vi "UHR-Fleezers Control (host) - 12.0.vi"() -> ()   [LabVIEW 2012] (continued)
        n1597 = case shown="True" w2753 {
          tunnel: [w2765 1] -> w2754
          tunnel: w2758 -> [w2767 _]
          tunnel: [w2766 w2785] -> w2755
          tunnel: w2756 -> [w2766 _]
          tunnel: w2752 -> [_ w2805]
          tunnel: w2745 -> [_ w2803]
          tunnel: w2747 -> [_ w2806]
          tunnel: [w2764 w2784] -> w2744
          tunnel: w2746 -> [w2764 _]
          tunnel: [w2763 w2782] -> w2741
          tunnel: w2742 -> [w2763 _]
          tunnel: [w2762 w2781] -> w2738
          tunnel: w2739 -> [w2762 _]
          tunnel: "Start Saving" -> [_ w2779]
          tunnel: w2734 -> [_ w2778]
          tunnel: [w2761 w2769] -> w2727
          tunnel: w2731 -> [w2761 _]
          tunnel: [w2760 w2768] -> w2728
          tunnel: w2729 -> [w2760 _]
          frame False {
            n1598 = Increment(x=w2767) -> (x+1=w2765:i32)
          }
          frame True {
            w2775 = FALSE ("Start Saving")
            w2780 = 9.0  # File Version
            w2788 = FALSE ("prepend array or string size? (T)")
            w2786 = T36."big-endian, network order" ("byte order (0:big-endian, network order)")
            n1599 = local read "BD 1 Frequency 1 (MHz)"() -> (w2802:dbl)
            n1600 = local read "BD 2 Frequency 1 (MHz)"() -> (w2801:dbl)
            n1601 = local read "BD 1 Frequency 2 (MHz)"() -> (w2800:dbl)
            n1602 = local read "BD 2 Frequency 2 (MHz)"() -> (w2799:dbl)
            n1603 = local read "BD 1 Frequency 3 (MHz)"() -> (w2798:dbl)
            n1604 = local read "BD 2 Frequency 3 (MHz)"() -> (w2797:dbl)
            n1605 = Array Size(array=w2778) -> (size(s)=w2777:i32)
            n1606 = To Double Precision Float(number=w2777) -> (double precision float=w2776:dbl)
            n1607 = local write "Save Calibration"(w2775) -> ()
            n1608 = local write "Start Saving"(w2775) -> ()
            n1609 = Build Array("Save APD Data\nwith Trap Data", "Save Trap Pos. Data") -> (w2772:bool[])
            n1610 = Boolean Array To Number(Boolean array=w2772) -> (number=w2771:u32)
            n1611 = Build Array(w2802, w2801, w2800, w2799, w2798, w2797) -> (w2796:dbl[])
            n1612 = case shown="1, Default" w2806 {
              tunnel: w2805 -> [w2877 w2897 w2913 w2951]
              tunnel: w2776 -> [w2882 w2904 w2933 w2970]
              tunnel: w2803 -> [w2881 w2903 w2932 w2969]
              tunnel: [w2878 w2899 w2924 w2961] -> w2794
              tunnel: [w2869 "Cal sets to save" w2914 w2952] -> w2784
              tunnel: w2796 -> [w2879 w2900 w2926 w2963]
              tunnel: "Save APD Data\nwith Trap Data" -> [w2876 _ w2910 w2949]
              tunnel: [w2876 w2891 w2910 w2949] -> w2781
              tunnel: w2780 -> [w2872 w2892 w2908 w2947]
              tunnel: w2779 -> [w2871 _ _ _]
              tunnel: [w2862 w2891 w2907 w2937] -> w2768
              tunnel: "Save Trap Pos. Data" -> [w2862 _ w2907 w2937]
              tunnel: w2771 -> [w2861 _ w2906 w2936]
              frame 1, Default {
                # "timeseries"
                n1613 = case shown="True" "Profile" {
                  tunnel: [w2885 w2889] -> w2866
                  tunnel: [w2885 w2888] -> w2865
                  tunnel: [w2885 w2887] -> w2864
                  tunnel: [w2885 w2886] -> w2863
                  frame False {
                    w2885 = 0.0 ("f")
                  }
                  frame True {
                    n1614 = local read "Current Position"() -> (w2890:cluster{dbl, dbl, dbl})
                    n1615 = local read "Y change (mm)"() -> (w2886:dbl)
                    n1616 = Unbundle(w2890) -> (w2889:dbl, w2888:dbl, w2887:dbl)
                  }
                }
                n1617 = local read "Save ave N"() -> (w2884:dbl)
                n1618 = Multiply(x=w2884, y=w2877) -> (x*y=w2883:dbl)
                n1619 = To Double Precision Float(number=w2861) -> (double precision float=w2875:dbl)
                n1620 = Build Array(w2872, w2877, w2883, w2882, w2881, 0.0 ("f")) -> (w2880:dbl[])
                n1621 = Build Array(w2875, w2866, w2865, w2864, w2863) -> (w2873:dbl[])
                n1622 = Select(t=u32 4000000000, s=w2871, f="N sets to save") -> (s? t:f=w2869:u32)
                n1623 = Build Array (concatenate)(w2880, w2879, w2873) -> (w2878:dbl[])
              }
              frame 2 {
                w2894 = 0.0 ("f")
                w2891 = FALSE ("Save APD Data\nwith Trap Data")
                # "calibration"
                n1624 = Boolean To (0,1)(Boolean=w2891) -> (0, 1=w2896:i16)
                n1625 = To Double Precision Float(number=w2896) -> (double precision float=w2895:dbl)
                n1626 = Build Array(w2895, w2894, w2894, w2894, w2894) -> (w2893:dbl[])
                n1627 = Build Array(w2892, w2897, w2897, w2904, w2903, 1.0 ("t")) -> (w2901:dbl[])
                n1628 = Build Array (concatenate)(w2901, w2900, w2893) -> (w2899:dbl[])
                "Calibrating Trap..." <- TRUE ("Calibrating...")
              }
              frame 4 {
                w2911 = 0.0 ("f")
                # "scan dir (x/y = 0/1)"
                # "cycles/step"
                # "n scans (f/b)"
                # "steps"
                # "freq. range"
                # "AOD raster scan"
                n1629 = local read "Number of F/B Scans (AOD)"() -> (w2918:u16)
                n1630 = local read "Cycles/step (AOD)"() -> (w2920:u64)
                n1631 = local read "Scan Range (MHz)"() -> (w2923:dbl)
                n1632 = local read "Scan steps (AOD)"() -> (w2922:u64)
                n1633 = local read "Scan BD"() -> (w2930:bool)
                n1634 = local read "Save ave N"() -> (w2935:dbl)
                n1635 = Boolean To (0,1)(Boolean=w2930) -> (0, 1=w2929:i16)
                n1636 = To Double Precision Float(number=w2918) -> (double precision float=w2917:dbl)
                n1637 = To Double Precision Float(number=w2922) -> (double precision float=w2921:dbl)
                n1638 = To Double Precision Float(number=w2920) -> (double precision float=w2919:dbl)
                n1639 = To Double Precision Float(number=w2929) -> (double precision float=w2928:dbl)
                n1640 = Multiply(x=w2935, y=w2913) -> (x*y=w2934:dbl)
                n1641 = To Double Precision Float(number=w2906) -> (double precision float=w2912:dbl)
                n1642 = Build Array(w2912, w2911, w2911, w2911, w2911) -> (w2909:dbl[])
                n1643 = local read "N sets should be saved"() -> (w2915:dbl)
                n1644 = Build Array(w2928, w2923, w2921, w2919, w2917) -> (w2925:dbl[])
                n1645 = Build Array(w2908, w2913, w2934, w2933, w2932, 2.0 ("t")) -> (w2927:dbl[])
                n1646 = Round Toward +Infinity(x=w2915) -> (ceil(x): smallest int >= x=w2916:dbl)
                n1647 = Build Array (concatenate)(w2927, w2926, w2909, w2925) -> (w2924:dbl[])
                n1648 = To Unsigned Long Integer(number=w2916) -> (unsigned 32bit integer=w2914:u32)
              }
              frame 8 {
                w2944 = 0.0 ("f")
                # "MCL raster scan"
                n1649 = local read "Number of scans (MCL)"() -> (w2939:u64)
                n1650 = local read "Scan lines (y)"() -> (w2938:u64)
                n1651 = local read "2D or 1D Scan"() -> (w2941:bool)
                n1652 = local read "Scan Range (V)\n(of steps)"() -> (w2960:dbl)
                n1653 = local read "Fast Scan Dir"() -> (w2967:bool)
                n1654 = local read "Cycles/step (MCL)"() -> (w2957:u64)
                n1655 = local read "Scan steps (MCL)"() -> (w2959:u64)
                n1656 = Select(t=w2938, s=w2941, f=w2939) -> (s? t:f=w2940:u64)
                n1657 = Boolean To (0,1)(Boolean=w2941) -> (0, 1=w2943:i16)
                n1658 = local read "Save ave N"() -> (w2972:dbl)
                n1659 = local read "Initial X"() -> (w2946:dbl)
                n1660 = local read "Initial Y"() -> (w2945:dbl)
                n1661 = To Double Precision Float(number=w2943) -> (double precision float=w2942:dbl)
                n1662 = Boolean To (0,1)(Boolean=w2967) -> (0, 1=w2966:i16)
                n1663 = To Double Precision Float(number=w2940) -> (double precision float=w2955:dbl)
                n1664 = To Double Precision Float(number=w2959) -> (double precision float=w2958:dbl)
                n1665 = To Double Precision Float(number=w2957) -> (double precision float=w2956:dbl)
                n1666 = To Double Precision Float(number=w2966) -> (double precision float=w2965:dbl)
                n1667 = Multiply(x=w2972, y=w2951) -> (x*y=w2971:dbl)
                n1668 = To Double Precision Float(number=w2936) -> (double precision float=w2950:dbl)
                n1669 = local read "N sets should be saved (MCL)"() -> (w2953:dbl)
                n1670 = Build Array(w2950, w2942, w2944, w2944, w2944) -> (w2948:dbl[])
                n1671 = Build Array(w2965, w2960, w2958, w2956, w2955, w2946, w2945) -> (w2962:dbl[])
                n1672 = Build Array(w2947, w2951, w2971, w2970, w2969, 3.0 ("t")) -> (w2964:dbl[])
                n1673 = Round Toward +Infinity(x=w2953) -> (ceil(x): smallest int >= x=w2954:dbl)
                n1674 = Build Array (concatenate)(w2964, w2963, w2948, w2962) -> (w2961:dbl[])
                n1675 = To Unsigned Long Integer(number=w2954) -> (unsigned 32bit integer=w2952:u32)
              }
            }
            n1676 = local read "Index"() -> (w2811:dbl)
            n1677 = call "Create new save file.vi"("Insert"="", "Ext"=".dat", "Index In"=w2811) -> ("Path Out"=w2770:path, "Index Out"=w2783:dbl)
            n1678 = local write "Save file name"(w2770) -> ()
            n1679 = local write "Index"(w2783) -> ()
            n1680 = local write "Save index"(w2783) -> ()
            n1681 = Array Size(array=w2794) -> (size(s)=w2795:i32)
            n1682 = Open/Create/Replace File(file path (use dialog)=w2770, operation (0:open)=T35."create", access (0:read/write)=enum16{"read/write", "read-only", "write-only"}."write-only") -> (refnum out=w2808:refnum<file>)  [unwired: 1 in, 4 out]
            n1683 = local write "Saving..."(TRUE ("Saving...")) -> ()
            n1684 = To Double Precision Float(number=w2795) -> (double precision float=w2793:dbl)
            n1685 = String Length(string="Comment (data description)") -> (length=w2791:i32)
            n1686 = To Double Precision Float(number=w2791) -> (double precision float=w2790:dbl)
            n1687 = Deny Access(7:w2808) -> (3:w2807:refnum<file>)  [unwired: 1 in, 2 out]
            n1688 = Build Array (concatenate)(w2793, w2794, w2790) -> (w2792:dbl[])
            n1689 = case "If fluorescence data to be saved" shown="True" w2781 {
              tunnel: w2770 -> [_ w2860]
              tunnel: [refnum<k0> refnum w2840] -> w2782
              frame False {
              }
              frame True {
                w2839 = 0.0
                n1690 = local read "APD Integration Time (s)"() -> (w2845:dbl)
                n1691 = local read "N APD Samp/step"() -> (w2838:dbl)
                n1692 = Path To String(path=w2860) -> (string=w2859:string)
                n1693 = String Length(string=w2859) -> (length=w2858:i32)
                n1694 = Subtract(x=w2858, y=4) -> (x-y=w2856:i32)
                n1695 = String Subset(string=w2859, length (rest)=w2856) -> (substring=w2855:string)  [unwired: 1 out]
                n1696 = Build Array(w2845, w2838, w2839, w2839, w2839, w2839, w2839, w2839) -> (w2842:dbl[])
                n1697 = Concatenate Strings(w2855, "_fl.dat" ("string")) -> (w2853:string)
                n1698 = Array Size(array=w2842) -> (size(s)=w2844:i32)
                n1699 = String To Path(string=w2853) -> (path=w2849:path)
                n1700 = Open/Create/Replace File(file path (use dialog)=w2849, operation (0:open)=T35."create", access (0:read/write)=enum16{"read/write", "read-only", "write-only"}."write-only") -> (refnum out=w2850:refnum<file>)  [unwired: 1 in, 4 out]
                n1701 = Deny Access(7:w2850) -> (3:w2846:refnum<file>)  [unwired: 1 in, 2 out]
                n1702 = To Double Precision Float(number=w2844) -> (double precision float=w2843:dbl)
                n1703 = Build Array (concatenate)(w2843, w2842) -> (w2841:dbl[])
                n1704 = Write to Binary File(file (use dialog)=w2846, data=w2841, 5:FALSE ("prepend array or string size? (T)"), 9:T36."big-endian, network order" ("byte order (0:big-endian, network order)")) -> (refnum out=w2840:refnum<file>)  [unwired: 1 in, 3 out]
              }
            }
            n1705 = case shown="True" w2768 {
              tunnel: w2770 -> [_ w2822]
              tunnel: [refnum<k0> refnum w2821] -> w2769
              frame False {
              }
              frame True {
                w2817 = 0.0 ("element")
                n1706 = Path To String(path=w2822) -> (string=w2836:string)
                n1707 = Build Array(w2817, w2817, w2817, w2817, w2817, w2817, w2817, w2817) -> (w2818:dbl[])
                n1708 = String Length(string=w2836) -> (length=w2835:i32)
                n1709 = Subtract(x=w2835, y=4) -> (x-y=w2833:i32)
                n1710 = Array Size(array=w2818) -> (size(s)=w2820:i32)
                n1711 = String Subset(string=w2836, length (rest)=w2833) -> (substring=w2832:string)  [unwired: 1 out]
                n1712 = To Double Precision Float(number=w2820) -> (double precision float=w2819:dbl)
                n1713 = Concatenate Strings(w2832, "_pos.dat" ("string")) -> (w2830:string)
                n1714 = Build Array (concatenate)(w2819, w2818) -> (w2816:dbl[])
                n1715 = String To Path(string=w2830) -> (path=w2826:path)
                n1716 = Open/Create/Replace File(file path (use dialog)=w2826, operation (0:open)=T35."create", access (0:read/write)=enum16{"read/write", "read-only", "write-only"}."write-only") -> (refnum out=w2827:refnum<file>)  [unwired: 1 in, 4 out]
                n1717 = Deny Access(7:w2827) -> (3:w2823:refnum<file>)  [unwired: 1 in, 2 out]
                n1718 = Write to Binary File(file (use dialog)=w2823, data=w2816, 5:FALSE ("prepend array or string size? (T)"), 9:T36."big-endian, network order" ("byte order (0:big-endian, network order)")) -> (refnum out=w2821:refnum<file>)  [unwired: 1 in, 3 out]
              }
            }
            n1719 = Write to Binary File(file (use dialog)=w2807, data=w2792, 5:w2788, 9:w2786) -> (refnum out=w2789:refnum<file>)  [unwired: 1 in, 3 out]
            n1720 = Write to Binary File(file (use dialog)=w2789, data="Comment (data description)", 5:w2788, 9:w2786) -> (refnum out=w2785:refnum<file>)  [unwired: 1 in, 3 out]
          }
        }
        n1721 = feedback-in #28(w2728) -> ()
        n1722 = feedback-in #29(w2755) -> ()
        n1723 = feedback-in #30(w2727) -> ()
        n1724 = feedback-in #31(w2738) -> ()
        n1725 = feedback-in #32(w2741) -> ()
        n1726 = feedback-in #33(w2754) -> ()
        n1727 = feedback-in #34(w2744) -> ()
      }
      frame #1 {
        n1728 = local read "Saving..."() -> (w2986:bool)
        n1729 = case shown="True" w2986 {
          tunnel: w2990 -> [_ w3001]
          tunnel: w2989 -> [_ w3015]
          tunnel: w2988 -> [_ w3011]
          tunnel: w2987 -> [_ w3010]
          tunnel: w2985 -> [_ w3009]
          tunnel: w2984 -> [_ w3004]
          tunnel: w2983 -> [_ w3003]
          tunnel: w2982 -> [_ w3002]
          tunnel: w2981 -> [_ w3000]
          tunnel: w2980 -> [_ w2998]
          tunnel: w2979 -> [_ w2997]
          tunnel: w2978 -> [_ w2996]
          tunnel: w2977 -> [_ w2995]
          tunnel: w2976 -> [_ w2994]
          tunnel: w2975 -> [_ w2993]
          tunnel: w2974 -> [_ w2992]
          tunnel: w2973 -> [_ w2991]
          frame False {
          }
          frame True {
            n1730 = Multiply(x=w3001, y=w3000) -> (x*y=→"Time (s)":dbl)
            n1731 = Less Or Equal?(x=w3001, y=w3009) -> (x <= y?=w3013:bool)
            n1732 = Or(x="Stop Saving", y="Abort save 2") -> (x .or. y?=w3005:bool)
            n1733 = Not(x=w3005) -> (.not. x?=w3014:bool)
            n1734 = And(x=w3013, y=w3014) -> (x .and. y?=w3012:bool)
            n1735 = case shown="True" w3012 {
              tunnel: w3015 -> [w3022 w3097]
              tunnel: [0.0 w3100] -> w3008
              tunnel: w3001 -> [_ w3098]
              tunnel: w3009 -> [_ w3099]
              tunnel: w3011 -> [_ w3094]
              tunnel: w3010 -> [_ _]
              tunnel: w3004 -> [w3020 w3087]
              tunnel: w3003 -> [w3019 w3088]
              tunnel: w3002 -> [_ w3086]
              tunnel: w2998 -> [_ w3085]
              tunnel: w2997 -> [_ w3029]
              tunnel: w2996 -> [_ w3078]
              tunnel: w2995 -> [_ w3056]
              tunnel: w2994 -> [w3016 w3038]
              tunnel: w2993 -> [w3017 w3037]
              tunnel: w2992 -> [_ w3034]
              tunnel: w2991 -> [_ w3032]
              frame False {
                w3018 = FALSE
                n1736 = Close File(refnum=w3022) -> ()  [unwired: 1 in, 2 out]
                n1737 = case shown="True" w3019 {
                  tunnel: w3020 -> [_ w3024]
                  frame False {
                  }
                  frame True {
                    n1738 = Close File(refnum=w3024) -> ()  [unwired: 1 in, 2 out]
                  }
                }
                n1739 = case shown="True" w3016 {
                  tunnel: w3017 -> [_ w3023]
                  frame False {
                  }
                  frame True {
                    n1740 = Close File(refnum=w3023) -> ()  [unwired: 1 in, 2 out]
                  }
                }
                n1741 = local write "Raster Scanning..."(w3018) -> ()
                n1742 = local write "Calibrating Trap..."(w3018) -> ()
                n1743 = call <vilib>:"Beep.vi"() -> ()  [unwired: 3 in, 9 out]
                n1744 = local write "Stop Saving"(w3018) -> ()
                "Saving..." <- w3018
              }
              frame True {
                n1745 = local read "Calibrating Trap..."() -> (w3089:bool)
                n1746 = case "Write fl. data" shown="True" w3088 {
                  tunnel: w3087 -> [_ w3123]
                  tunnel: w3086 -> [_ w3122]
                  frame False {
                  }
                  frame True {
                    n1747 = Write to Binary File(file (use dialog)=w3123, data=w3122, 5:FALSE ("prepend array or string size? (T)"), 9:T36."big-endian, network order" ("byte order (0:big-endian, network order)")) -> ()  [unwired: 1 in, 4 out]
                  }
                }
                n1748 = Greater?(x="Save ave N", y=1.0) -> (0:w3092:bool)
                n1749 = Not(x=w3089) -> (.not. x?=w3091:bool)
                n1750 = And(x=w3091, y=w3092) -> (x .and. y?=w3035:bool)
                n1751 = case shown="True" w3035 {
                  tunnel: w3034 -> [w3103 w3114]
                  tunnel: [w3103 w3106] -> w3033
                  tunnel: "Save ave N" -> [_ w3107]
                  frame False {
                  }
                  frame True {
                    w3104 = 2 ("dimension size")
                    n1752 = Array Size(array=w3114) -> (size(s)=w3108:i32)
                    n1753 = Divide(x=w3108, y=w3104) -> (x/y=w3112:dbl)
                    n1754 = Reshape Array(w3114, w3112, w3104) -> (w3113:u64[][])
                    n1755 = Transpose 2D Array(2D array=w3113) -> (transposed array=w3111:u64[][])
                    n1756 = for {
                      tunnel: w3111 -> [w3116] mode=indexing
                      tunnel: [w3115] -> w3105 mode=indexing
                      tunnel: w3107 -> [w3117]
                      workers-P: _ -> [_]
                      n1757 = call "downsample 1D array - U64.vi"("Ave N"=w3117, "Array In"=w3116) -> ("Array Out"=w3115:u64[])  [unwired: 1 in]
                    }
                    n1758 = Transpose 2D Array(2D array=w3105) -> (transposed array=w3110:u64[][])
                    n1759 = Divide(x=w3108, y=w3107) -> (x/y=w3109:dbl)
                    n1760 = Reshape Array(w3110, w3109) -> (w3106:u64[])
                  }
                }
                n1761 = case shown="True" w3035 {
                  tunnel: w3094 -> [w3126 w3138]
                  tunnel: [w3126 w3130] -> w3090
                  tunnel: "Save ave N" -> [_ w3131]
                  tunnel: w3085 -> [_ w3129]
                  frame False {
                  }
                  frame True {
                    n1762 = Array Size(array=w3138) -> (size(s)=w3132:i32)
                    n1763 = Array Size(array=w3129) -> (size(s)=w3128:i32)
                    n1764 = Divide(x=w3132, y=w3128) -> (x/y=w3136:dbl)
                    n1765 = Reshape Array(w3138, w3136, w3128) -> (w3137:i16[][])
                    n1766 = Transpose 2D Array(2D array=w3137) -> (transposed array=w3135:i16[][])
                    n1767 = for {
                      tunnel: w3135 -> [w3141] mode=indexing
                      tunnel: [w3140] -> w3127 mode=indexing
                      tunnel: w3131 -> [w3139]
                      workers-P: _ -> [_]
                      n1768 = call "downsample 1D array - I16.vi"("Ave N"=w3139, "Array In"=w3141) -> ("Array Out"=w3140:i16[])  [unwired: 1 out]
                    }
                    n1769 = Transpose 2D Array(2D array=w3127) -> (transposed array=w3134:i16[][])
                    n1770 = Divide(x=w3132, y=w3131) -> (x/y=w3133:dbl)
                    n1771 = Reshape Array(w3134, w3133) -> (w3130:i16[])
                  }
                }
                n1772 = Index Array(array=w3056, index=1) -> (element=w3059:waveform(dbl))
                n1773 = Index Array(array=w3056, index=0) -> (element=w3061:waveform(dbl))
                n1774 = Unbundle By Name(w3059) -> ("Y"=w3063:dbl[])
                n1775 = Unbundle By Name(w3061) -> ("Y"=w3071:dbl[])
                n1776 = case "Write trap pos. data" shown="True" w3038 {
                  tunnel: w3037 -> [_ w3119]
                  tunnel: w3033 -> [_ w3118]
                  frame False {
                  }
                  frame True {
                    n1777 = Write to Binary File(file (use dialog)=w3119, data=w3118, 5:FALSE ("prepend array or string size? (T)"), 9:T36."big-endian, network order" ("byte order (0:big-endian, network order)")) -> ()  [unwired: 1 in, 4 out]
                  }
                }
                n1778 = Write to Binary File(file (use dialog)=w3097, data=w3090, 5:FALSE ("prepend array or string size? (T)"), 9:T36."big-endian, network order" ("byte order (0:big-endian, network order)")) -> ()  [unwired: 1 in, 4 out]
                n1779 = feedback #35(w3063) -> (w3065:dbl[])
                n1780 = Build Array (concatenate)(w3065, w3063) -> (w3064:dbl[])
                n1781 = Select(t=w3063, s=w3029, f=w3064) -> (s? t:f=w3049:dbl[])
                n1782 = feedback-in #35(w3049) -> ()
                n1783 = feedback #36(w3071) -> (w3084:dbl[])
                n1784 = Build Array (concatenate)(w3084, w3071) -> (w3083:dbl[])
                n1785 = Select(t=w3071, s=w3029, f=w3083) -> (s? t:f=w3058:dbl[])
                n1786 = feedback-in #36(w3058) -> ()
                n1787 = Divide(x=w3098, y=w3099) -> (x/y=w3101:dbl)
                n1788 = Multiply(x=w3101, y=100.0) -> (x*y=w3100:dbl)
                n1789 = Build Array(w3058, w3049) -> (→"Saved APD":dbl[][])
                n1790 = Array Size(array=w3058) -> (size(s)=w3076:i32)
                n1791 = Unbundle By Name(w3078) -> ("Y"=w3082:dbl[])
                n1792 = Subtract(x=w3076, y="N pts to average") -> (x-y=w3052:i32)
                n1793 = Multiply(x="N pts to average", y=u16 2) -> (x*y=w3053:u16)
                n1794 = Subtract(x=w3076, y=w3053) -> (x-y=w3051:i32)
                n1795 = feedback #37(w3082) -> (w3081:dbl[])
                n1796 = Build Array (concatenate)(w3081, w3082) -> (w3080:dbl[])
                n1797 = Select(t=w3082, s=w3029, f=w3080) -> (s? t:f=w3079:dbl[])
                "Trap Delta Graph" <- w3079
                n1798 = feedback-in #37(w3079) -> ()
                n1799 = Array Subset(array=w3058, index=w3052, length="N pts to average") -> (w3075:dbl[])
                n1800 = Array Subset(array=w3058, index=w3051, length="N pts to average") -> (w3074:dbl[])
                n1801 = Array Subset(array=w3049, index=w3052, length="N pts to average") -> (w3055:dbl[])
                n1802 = Array Subset(array=w3049, index=w3051, length="N pts to average") -> (w3054:dbl[])
                n1803 = Index Array(array=w3032, index=0) -> (element=w3030:waveform(dbl))
                n1804 = call-poly <vilib>:"Mean.vi"("X"=w3075) -> ("mean"=w3073:dbl)  [unwired: 1 out]
                n1805 = call-poly <vilib>:"Mean.vi"("X"=w3055) -> ("mean"=w3048:dbl)  [unwired: 1 out]
                n1806 = call-poly <vilib>:"Mean.vi"("X"=w3074) -> ("mean"=w3072:dbl)  [unwired: 1 out]
                n1807 = call-poly <vilib>:"Mean.vi"("X"=w3054) -> ("mean"=w3047:dbl)  [unwired: 1 out]
                n1808 = Unbundle By Name(w3030) -> ("Y"=w3027:dbl[])
                n1809 = Subtract(x=w3048, y=w3047) -> (x-y=w3039:dbl)
                "Delta Fl. 2" <- w3039
                n1810 = Subtract(x=w3073, y=w3072) -> (x-y=w3070:dbl)
                "Delta Fl. 1" <- w3070
                n1811 = Initialize Array(w3070, 1 ("dimension size")) -> (w3067:dbl[])
                n1812 = Initialize Array(w3039, 1 ("dimension size")) -> (w3044:dbl[])
                n1813 = feedback #38(w3067) -> (w3068:dbl[])
                n1814 = Build Array (concatenate)(w3068, w3067) -> (w3066:dbl[])
                n1815 = feedback #39(w3044) -> (w3045:dbl[])
                n1816 = Build Array (concatenate)(w3045, w3044) -> (w3043:dbl[])
                n1817 = feedback #40(w3027) -> (w3026:dbl[])
                n1818 = Build Array (concatenate)(w3026, w3027) -> (w3028:dbl[])
                n1819 = Select(t=w3027, s=w3029, f=w3028) -> (s? t:f=w3025:dbl[])
                "Saved trap pos" <- w3025
                n1820 = feedback-in #40(w3025) -> ()
                n1821 = Select(t=w3067, s=w3029, f=w3066) -> (s? t:f=w3042:dbl[])
                n1822 = feedback-in #38(w3042) -> ()
                n1823 = Select(t=w3044, s=w3029, f=w3043) -> (s? t:f=w3041:dbl[])
                n1824 = feedback-in #39(w3041) -> ()
                n1825 = Build Array(w3042, w3041) -> (→"Save APD Deriv":dbl[][])
              }
            }
            "Progress" <- w3008
            "Progress 2" <- w3008
          }
        }
      }
    }
    n1826 = local read "wait to reset values"() -> (w1737:bool)
    n1827 = Not(x=w1735) -> (.not. x?=w1738:bool)
    n1828 = And(x=w1738, y=w1737) -> (x .and. y?=w1739:bool)
    n1829 = case "Part of MCL raster scanning: returns to initial positions after scan done" shown="True" w1739 {
      tunnel: w1460 -> [w2548 w2555]
      tunnel: [w2548 w2554] -> w1741
      tunnel: w1459 -> [w2547 w2553]
      tunnel: [w2547 w2552] -> w1736
      frame False {
      }
      frame True {
        w2563 = 10.0 ("y")
        w2562 = 32767.0 ("y")
        # "to return scan values\nafter a synchronous \nAOM scan"
        n1830 = local read "AO2"() -> (w2556:dbl)
        n1831 = local read "AO1"() -> (w2557:dbl)
        n1832 = local write "wait to reset values"(FALSE ("wait to reset values")) -> ()
        n1833 = Multiply(x=w2557, y=w2562) -> (x*y=w2559:dbl)
        n1834 = Multiply(x=w2556, y=w2562) -> (x*y=w2561:dbl)
        n1835 = Divide(x=w2559, y=w2563) -> (x/y=w2558:dbl)
        n1836 = Divide(x=w2561, y=w2563) -> (x/y=w2560:dbl)
        n1837 = To Word Integer(number=w2558) -> (16bit integer=w2564:i16)
        n1838 = To Word Integer(number=w2560) -> (16bit integer=w2565:i16)
        n1839 = local read "Total Counts (ticks)"() -> (w2549:u32)
        n1840 = xnode "Read/Write Control"("FPGA VI Reference In"=w2555, "error in"=w2553, "AO1"=w2564, "AO2"=w2565, "MCL count"=w2549) -> ("FPGA VI Reference Out"=w2554:T19, "error out"=w2552:errorcluster)
        n1841 = local read "Scan Range (V)\n(of steps)"() -> (w2550:dbl)
        n1842 = property on="Scan Range (V)\n(of steps)" class="DigNum (strict)"("Val(Sgnl)"=w2550) -> ()  [unwired: 2 in, 2 out]
      }
    }
    n1843 = node-c288() -> ()  [unwired: 2 out]
  }
  n1844 = timed-loop "Control parameters (event loop)" {
    tunnel: w6 -> [w3150]
    shift-right: [w3149] -> _
    shift-left: errorcluster {"status"=FALSE, "code"=0, "source"=""} ("error out") -> [w3148]
    tunnel: [w3147] -> _
    timing: w97 -> [_]
    timing-out: [_] -> w96
    tunnel: w69 -> [w3146]
    tunnel: w10 -> [w3145]
    tunnel: w9 -> [w3144]
    tunnel: w8 -> [w3143]
    tunnel: w7 -> [w3142]
    stop <- w3147 stop-if-true
    n1845 = node-c288() -> ()  [unwired: 2 out]
    n1846 = event shown="[30] \"Invert APD Gate\", \"APD Gate ON Count\", \"APD Gate OFF Count\", \"APD Gate\", \"APD Integration Time (s)\", \"APD 1 AO Mult.\", \"APD 2 AO Mult.\", \"On one out of X cycles\": Value Change" {
      selector: _ -> [_ _ _ _ _ _ _ _ _ _ _ _ _ _ _ _ _ _ _ _ _ _ _ _ _ _ _ _ _ _ _ _ _ _ _ _ _ _ _ _ _ _ _ _ _ _ _ _ _ _ _ _ _ _ _ _ _ _ _ _ _ _ _ _ _ _ _ _ _ _ _ _ _ _ _ _]
      dyn-events: _ -> [_ _ _ _ _ _ _ _ _ _ _ _ _ _ _ _ _ _ _ _ _ _ _ _ _ _ _ _ _ _ _ _ _ _ _ _ _ _ _ _ _ _ _ _ _ _ _ _ _ _ _ _ _ _ _ _ _ _ _ _ _ _ _ _ _ _ _ _ _ _ _ _ _ _ _ _]
      timeout: _ -> [_ _ _ _ _ _ _ _ _ _ _ _ _ _ _ _ _ _ _ _ _ _ _ _ _ _ _ _ _ _ _ _ _ _ _ _ _ _ _ _ _ _ _ _ _ _ _ _ _ _ _ _ _ _ _ _ _ _ _ _ _ _ _ _ _ _ _ _ _ _ _ _ _ _ _ _]
      tunnel: w3150 -> [w3188 _ _ _ w3226 _ w3248 _ _ _ _ w3314 _ _ w3357 w3363 w3368 w3374 w3410 w3428 w3435 _ w3447 w3451 w3462 w3473 w3484 w3495 w3506 w3517 w3544 w3638 w3645 w3683 _ w3718 w3722 w3733 w3737 w3741 _ w3749 _ _ _ _ _ _ _ _ _ _ _ _ _ _ _ _ _ w4127 _ w4144 _ w4151 w4169 _ w4176 w4184 w4199 w4210 w4216 _ w4225 _ w4244 _]
      tunnel: [w3187 _ _ _ w3216 _ w3247 _ _ w3279 _ w3293 _ _ w3356 w3359 w3365 w3371 w3409 w3426 w3434 _ w3445 _ w3456 w3467 w3478 w3489 w3500 w3511 w3542 w3636 w3643 w3681 _ w3716 w3720 w3723 w3735 w3739 _ w3747 _ _ _ _ _ _ _ _ _ _ _ _ _ _ _ _ _ w4125 _ _ _ _ w4166 _ _ _ _ _ _ _ _ _ _ _] -> w3149
      tunnel: w3148 -> [w3186 _ _ _ w3225 _ w3246 _ _ w3279 _ w3313 _ _ w3355 w3358 w3364 w3370 w3408 w3427 w3433 _ w3446 w3450 w3461 w3472 w3483 w3494 w3505 w3516 w3543 w3637 w3644 w3682 _ w3717 w3721 w3732 w3736 w3740 _ w3748 _ _ _ _ _ _ _ _ _ _ _ _ _ _ _ _ _ w4126 _ w4143 _ w4150 w4168 _ w4175 w4183 w4198 w4209 w4215 _ w4224 _ w4243 _]
      tunnel: [_ _ _ _ _ _ _ _ _ w3278 _ _ _ _ _ _ _ _ _ _ _ _ _ _ _ _ _ _ _ _ _ _ _ _ _ _ _ _ _ _ _ _ _ _ _ _ _ _ _ _ _ _ _ _ _ _ _ _ _ _ _ _ _ _ _ _ _ _ _ _ _ _ _ _ _ _] -> w3147
      tunnel: [_ _ _ _ _ _ _ "Round T1 X" _ _ _ _ _ _ _ _ _ _ _ _ _ _ _ _ _ _ _ _ _ _ _ _ _ _ _ _ _ _ _ _ _ _ _ _ _ _ _ _ _ _ _ _ _ _ _ _ _ _ _ _ _ _ _ _ _ _ _ _ _ _ _ _ _ _ _ _] -> _
      tunnel: [_ _ _ "Adjust Scale\nto Mean" _ _ _ _ _ _ _ _ _ _ _ _ _ _ _ _ _ _ "Test ttrig" _ _ _ _ _ _ _ _ _ _ _ _ _ _ _ _ _ _ _ _ _ _ _ _ _ _ "Flush Sample" "Flush Pump 3" "Flush Pump 1" "Clear Volume" _ _ _ _ _ _ _ _ _ _ _ _ _ _ _ _ _ _ _ _ _ _ _] -> _
      tunnel: [_ _ _ _ _ _ _ _ "Round T2 X" _ "Delayed Interlace Start" _ _ _ _ _ _ _ _ _ _ _ _ _ _ _ _ _ _ _ _ _ _ _ _ _ _ _ _ _ _ _ _ _ _ _ _ _ _ _ _ _ _ _ _ _ _ _ _ _ _ _ _ _ _ _ _ _ _ _ _ _ _ _ _ _] -> _
      tunnel: w3146 -> [_ _ _ _ _ _ _ _ _ _ _ _ _ _ _ _ _ _ _ _ _ _ _ _ _ _ _ _ _ _ _ _ _ _ _ _ _ _ _ _ _ _ _ _ _ w3906 w3913 w3920 w3925 w3934 _ _ w4040 _ _ _ _ _ _ _ _ _ _ _ _ _ _ _ _ _ _ _ _ _ _ _]
      tunnel: w3145 -> [_ _ _ _ _ _ _ _ _ _ _ _ _ _ _ _ _ _ _ _ _ _ _ _ _ _ _ _ _ _ _ _ _ _ _ _ _ _ _ _ _ _ _ w3823 _ _ _ _ _ _ w3978 _ _ w4046 _ w4055 _ w4069 _ _ _ _ _ _ _ _ _ _ _ _ _ _ _ _ _ _]
      tunnel: w3144 -> [_ _ _ _ _ _ _ _ _ _ _ _ _ _ _ _ _ _ _ _ _ _ _ _ _ _ _ _ _ _ _ _ _ _ _ _ _ _ _ _ _ _ _ _ _ _ _ _ _ _ _ _ _ _ _ _ _ _ _ _ _ _ _ _ _ _ _ _ _ _ _ _ _ _ _ _]
      tunnel: w3143 -> [_ _ _ _ _ _ _ _ _ _ _ _ _ _ _ _ _ _ _ _ _ _ _ _ _ _ _ _ _ _ _ _ _ _ _ _ _ _ _ _ _ _ w3760 _ _ _ _ _ _ _ _ w4008 _ _ w4051 _ w4062 _ w4094 _ _ _ _ _ _ _ _ _ _ _ _ _ _ _ _ _]
      tunnel: w3142 -> [_ _ _ _ _ _ _ _ _ _ _ _ _ _ _ _ _ _ _ _ _ _ _ _ _ _ _ _ _ _ _ _ _ _ _ _ _ _ _ _ _ _ _ _ _ _ _ _ _ _ _ _ _ _ _ _ _ _ _ _ _ _ _ _ _ _ _ _ _ _ _ _ _ _ _ _]
      event "AI Count (ticks)", "Sets to FIFO (Traps)", "Save ave N", "FPGA Ave.", "# Samples/channel", "N sets to save": Value Change {
        # "So that if 'Save ave N' is updated, the AOD scanning code updates too."
        n1847 = event-data() -> ()  [unwired: 6 out]
        n1848 = local read "AI Count (ticks)"() -> (w3168:u32)
        n1849 = Boolean To (0,1)(Boolean="Sets to FIFO (Traps)") -> (0, 1=w3178:cluster{"Set 1":i16, "Set 2":i16, "Set 3":i16})
        n1850 = xnode "Read/Write Control"("FPGA VI Reference In"=w3188, "error in"=w3186, "ai count"=w3168, "AI1 Sets to FIFO"="Sets to FIFO (Traps)", "N of AI1 Int Acq Sets"="N Acq Sets (Traps + Fl.)") -> ("error out"=w3187:errorcluster)  [unwired: 1 out]
        n1851 = Cluster To Array(cluster=w3178) -> (array=w3177:i16[])
        n1852 = To Unsigned Long Integer(number=w3177) -> (unsigned 32bit integer=w3157:u32[])
        n1853 = local read "Scan steps (AOD)"() -> (w3179:u64)
        n1854 = Multiply(x=w3168, y="N Acq Sets (Traps + Fl.)") -> (x*y=w3166:u32)
        n1855 = Divide(x=40000000.0, y=w3168) -> (x/y=w3160:dbl)
        "AI rate (Hz)" <- w3160
        "Ave. Rate (Hz)" <- w3160
        n1856 = Add Array Elements(numeric array=w3157) -> (sum=w3169:u32)
        "Trap Sets" <- w3169
        n1857 = Reciprocal(x=w3160) -> (1/x=→"Ave. Period (s)":dbl)
        n1858 = property on="Scan steps (AOD)" class="DigNum (strict)"("Val(Sgnl)"=w3179) -> ()  [unwired: 2 in, 2 out]
        n1859 = Divide(x=w3160, y="N Acq Sets (Traps + Fl.)") -> (x/y=w3183:dbl)
        "Data Rate (Hz)" <- w3183
        n1860 = Reciprocal(x=w3183) -> (1/x=→"Data Period (s)":dbl)
        n1861 = local read "Save ave N"() -> (w3182:dbl)
        n1862 = Divide(x=w3183, y=w3182) -> (x/y=w3181:dbl)
        "Save Data Rate (Hz)" <- w3181
        n1863 = Reciprocal(x=w3181) -> (1/x=→"Save Data Period (s)":dbl)
        n1864 = Multiply(x=w3166, y="# Samples/trap") -> (x*y=w3164:u32)
        "Counts/DMA" <- w3164
        n1865 = property on="Trap Disp. Downsample" class="DigNum (strict)"("Maximum"="# Samples/trap") -> ()  [unwired: 2 in, 2 out]
        n1866 = Multiply(x=w3169, y="# Samples/trap") -> (x*y=w3158:u32)
        "# Samples/channel" <- w3158
        n1867 = Multiply(x=w3158, y=u32 8) -> (x*y=→"Trap AI Elements/DMA read":u32)
        n1868 = local read "APD Int. Count"() -> (w3165:u32)
        n1869 = Multiply(x=w3158, y=u32 3) -> (x*y=→"Trap Pos Elements/DMA read":u32)
        n1870 = Divide(x=w3164, y=w3165) -> (x/y=w3155:dbl)
        "APD Samples/FIFO Acq." <- w3155
        n1871 = Divide(x=w3164, y=40000000.0) -> (x/y=w3162:dbl)
        "DMA Update Period (s)" <- w3162
        n1872 = Multiply(x=2.0, y=w3155) -> (x*y=→"APD Elements/DMA read":dbl)
        n1873 = property on="APD Disp. Downsample" class="DigNum (strict)"("Maximum"=w3155) -> ()  [unwired: 2 in, 2 out]
        n1874 = local read "N sets to save"() -> (w3175:u32)
        n1875 = Multiply(x=w3162, y=w3175) -> (x*y=→"Total Time (s)":dbl)
        "FPGA Averaging" <- FALSE ("FPGA Averaging")
      }
      event "Remove Offset": Value Change {
        n1876 = event-data() -> ()  [unwired: 7 out]
        n1877 = local write "Remove Offset"(FALSE ("Remove Offset")) -> ()
        n1878 = local read "Bead Mean (nm)"() -> (w3190:dbl)
        n1879 = local read "Offset (nm)"() -> (w3191:dbl)
        n1880 = Add(x=w3190, y=w3191) -> (x+y=w3189:dbl)
        n1881 = local write "Offset (nm)"(w3189) -> ()
        n1882 = disable-structure shown="Disabled" {
          frame Disabled {
            n1883 = local read "Bead Mean (nm)"() -> (w3196:dbl)
            n1884 = Add(y=w3196) -> (x=w3195:dbl, x+y=w3194:dbl)
            n1885 = Subtract(x=w3196, y=w3195) -> (x-y=w3193:dbl)
            n1886 = property on="Bead Separation" class="WFChart (strict)"("YScale.Minimum"=w3193) -> ()  [unwired: 2 in, 2 out]
            n1887 = property on="Bead Separation" class="WFChart (strict)"("YScale.Maximum"=w3194) -> ()  [unwired: 2 in, 2 out]
          }
          frame Enabled {
          }
        }
      }
      event "Detector Type": Value Change {
        n1888 = event-data() -> ()  [unwired: 7 out]
        n1889 = local read "AI labels"() -> (w3197:string[])
        n1890 = property on="High Res. Display" class="Ring (strict)"("Strings []"=w3197) -> ()  [unwired: 2 in, 2 out]
        n1891 = Build Array (concatenate)(w3197, "none") -> (w3198:string[])
        n1892 = property on="FFT 1 Choice 1" class="Ring (strict)"("Strings []"=w3198) -> ()  [unwired: 2 in, 2 out]
        n1893 = property on="FFT 1 Choice 2" class="Ring (strict)"("Strings []"=w3198) -> ()  [unwired: 2 in, 2 out]
        n1894 = property on="FFT 2 Choice 1" class="Ring (strict)"("Strings []"=w3198) -> ()  [unwired: 2 in, 2 out]
        n1895 = property on="FFT 2 Choice 2" class="Ring (strict)"("Strings []"=w3198) -> ()  [unwired: 2 in, 2 out]
        n1896 = Bundle("APD 1", "APD 2") -> (w3201:cluster{string, string})  [unwired: 1 out]
        n1897 = Cluster To Array(cluster=w3201) -> (array=w3199:string[])
        n1898 = Build Array (concatenate)(w3199, w3198) -> (w3203:string[])
        n1899 = Array Size(array=w3203) -> (size(s)=w3204:i32)
        n1900 = property on="Signals to Plot" class="LstBox (strict)"("Item Names"=w3203) -> ()  [unwired: 2 in, 2 out]
        n1901 = property on="Signals to Plot" class="LstBox (strict)"("Number of Rows"=w3204) -> ()  [unwired: 2 in, 2 out]
        n1902 = property on="All Signals" class="WFChart (strict)"("LegNumRows"=w3204) -> ()  [unwired: 2 in, 2 out]
      }
      event "Adjust Scale\nto Mean": Value Change {
        n1903 = event-data() -> ()  [unwired: 7 out]
        n1904 = local read "APD 1 Rate (Hz)"() -> (w3213:dbl)
        n1905 = Multiply(x=1000.0, y="Above (kHz)") -> (x*y=w3211:dbl)
        n1906 = Multiply(x=1000.0, y="Below (kHz)") -> (x*y=w3209:dbl)
        n1907 = Add(x=w3211, y=w3213) -> (x+y=w3206:dbl)
        n1908 = Subtract(x=w3213, y=w3209) -> (x-y=w3207:dbl)
        n1909 = property on="APD Chart" class="WFChart (strict)"("YScale.Minimum"=w3207) -> ()  [unwired: 2 in, 2 out]
        n1910 = property on="APD Chart" class="WFChart (strict)"("YScale.Maximum"=w3206) -> ()  [unwired: 2 in, 2 out]
      }
      event "Phase adj. (AI1)", "+ phase (AI1)", "- phase (AI1)": Value Change {
        n1911 = event-data() -> ()  [unwired: 7 out]
        n1912 = Negate(x="Phase adj. (AI1)") -> (-x=w3223:i16)
        n1913 = Select(t=w3223, s="- phase (AI1)", f="Phase adj. (AI1)") -> (s? t:f=w3222:i16)
        n1914 = xnode "Read/Write Control"("FPGA VI Reference In"=w3226, "error in"=w3225, "Phase count adjustment"=w3222) -> ("FPGA VI Reference Out"=w3221:T19, "error out"=w3220:errorcluster)
        n1915 = Or(x="- phase (AI1)", y="+ phase (AI1)") -> (x .or. y?=w3217:bool)
        n1916 = xnode "Read/Write Control"("FPGA VI Reference In"=w3221, "error in"=w3220, "+ phase"=w3217) -> ("error out"=w3216:errorcluster)  [unwired: 1 out]
      }
      event "Signals to Plot": Double Click {
        w3229 = u32 9868950 ("Color Box")
        n1917 = event-data() -> ("Row"=w3231:i32)  [unwired: 9 out]
        n1918 = property on="All Signals" class="WFChart (strict)"("Active Plot"=w3231) -> (error out=w3242:errorcluster)  [unwired: 2 in, 1 out]
        n1919 = property on="All Signals" class="WFChart (strict)" props=["Plot", "Visible?", "Plot", "Plot Color"](error in=w3242) -> (error out=w3241:errorcluster, "Plot.Visible?"=w3240:bool)  [unwired: 1 in, 2 out]
        n1920 = Select(t=FALSE ("Plot.Visible"), s=w3240, f=TRUE ("Plot.Visible")) -> (s? t:f=w3235:bool)
        n1921 = property on="All Signals" class="WFChart (strict)"(error in=w3241, "Plot.Visible?"=w3235) -> (error out=w3237:errorcluster)  [unwired: 1 in, 1 out]
        n1922 = property on="All Signals" class="WFChart (strict)"(error in=w3237) -> (error out=w3232:errorcluster, "Plot.Plot Color"=w3236:u32)  [unwired: 1 in, 1 out]
        n1923 = property on="Signals to Plot" class="LstBox (strict)"(error in=w3232, "Active Row"=w3231) -> (error out=w3230:errorcluster)  [unwired: 1 in, 1 out]
        n1924 = Select(t=w3236, s=w3235, f=u32 0) -> (s? t:f=w3233:u32)
        n1925 = property on="Signals to Plot" class="LstBox (strict)"(error in=w3230, "CellFontColor"=w3233, "SelColor"=w3229, "CellBG"=w3229, "CellFontSize"=u32 20 ("Active Row:Cell Font:Size"), "CellFontBold"=TRUE ("Active Row:Cell Font:Bold")) -> ()  [unwired: 1 in, 2 out]
      }
      event "BD 1 Frequency 1 (MHz)", "BD 1 Frequency 2 (MHz)", "BD 1 Frequency 3 (MHz)", "BD 2 Frequency 1 (MHz)", "BD 2 Frequency 2 (MHz)", "BD 2 Frequency 3 (MHz)", "Trap Delta (MHz)": Value Change {
        n1926 = event-data() -> ("CtlRef"=w3245:refnum<vi>)  [unwired: 6 out]
        n1927 = control-ref of="Trap Delta (MHz)"() -> (w3244:refnum<vi>)
        n1928 = Equal?(x=w3244, y=w3245) -> (x = y?=w3243:bool)
        n1929 = case shown="False" "Oscillate Set 1" {
          tunnel: w3248 -> [w3268 _]
          tunnel: [w3267 w3271] -> w3247
          tunnel: w3246 -> [w3266 w3271]
          tunnel: w3243 -> [w3251 _]
          frame False {
            n1930 = local read "BD 1 Frequency 2 (MHz)"() -> (w3255:dbl)
            n1931 = local read "BD 1 Frequency 1 (MHz)"() -> (w3253:dbl)
            n1932 = Subtract(x=w3255, y="Trap Delta (MHz)") -> (x-y=w3252:dbl)
            n1933 = Select(t=w3252, s=w3251, f=w3253) -> (s? t:f=w3250:dbl)
            n1934 = local read "Y RF Frequency Limits (MHz)"() -> (w3256:T16)
            n1935 = local read "X RF Frequency Limits (MHz)"() -> (w3257:T16)
            n1936 = local read "BD 1 Frequency 3 (MHz)"() -> (w3269:dbl)
            n1937 = local write "BD 1 Frequency 1 (MHz)"(w3250) -> ()
            n1938 = local read "BD 2 Frequency 1 (MHz)"() -> (w3260:dbl)
            n1939 = local read "BD 2 Frequency 2 (MHz)"() -> (w3259:dbl)
            n1940 = local read "BD 2 Frequency 3 (MHz)"() -> (w3270:dbl)
            n1941 = call "set RF board frequency - interlace.vi"("Board 2 Frequency Limits"=w3256, "Board 1 Frequency Limits"=w3257, "error in"=w3266, "FPGA VI Reference In"=w3268, "Board 2 Frequency 3 (MHz)"=w3270, "Board 1 Frequency 3 (MHz)"=w3269, "Board 2 Frequency 2 (MHz)"=w3259, "Board 2 Frequency 1 (MHz)"=w3260, "Board 1 Frequency 2 (MHz)"=w3255, "Board 1 Frequency 1  (MHz)"=w3250) -> ("error out"=w3267:errorcluster)  [unwired: 1 out]
            n1942 = Subtract(x=w3260, y=w3259) -> (x-y=w3264:dbl)
            n1943 = Subtract(x=w3250, y=w3255) -> (x-y=w3265:dbl)
            n1944 = Square(x=w3264) -> (x^2=w3262:dbl)
            n1945 = Square(x=w3265) -> (x^2=w3263:dbl)
            n1946 = Add(x=w3263, y=w3262) -> (x+y=w3261:dbl)
            n1947 = Square Root(x=w3261) -> (sqrt(x)=w3258:dbl)
            n1948 = local write "Trap Delta (MHz)"(w3258) -> ()
            n1949 = property on="Initial delta (MHz)" class="DigNum (strict)"("Val(Sgnl)"=w3258) -> ()  [unwired: 2 in, 2 out]
          }
          frame True {
          }
        }
      }
      event "Round T1 X": Value Change {
        n1950 = event-data() -> ()  [unwired: 7 out]
        n1951 = local read "BD 1 Frequency 1 (MHz)"() -> (w3274:dbl)
        n1952 = Round To Nearest(number=w3274) -> (nearest integer value=w3273:dbl)
        n1953 = property on="BD 1 Frequency 1 (MHz)" class="DigNum (strict)"("Val(Sgnl)"=w3273) -> ()  [unwired: 2 in, 2 out]
      }
      event "Round T2 X": Value Change {
        n1954 = event-data() -> ()  [unwired: 7 out]
        n1955 = local read "BD 1 Frequency 2 (MHz)"() -> (w3276:dbl)
        n1956 = Round To Nearest(number=w3276) -> (nearest integer value=w3275:dbl)
        n1957 = property on="BD 1 Frequency 2 (MHz)" class="DigNum (strict)"("Val(Sgnl)"=w3275) -> ()  [unwired: 2 in, 2 out]
      }
      event "Stop All": Value Change {
        n1958 = event-data() -> ()  [unwired: 7 out]
        n1959 = local read "Stop All"() -> (w3278:bool)
      }
      event "Delayed Interlace Start": Value Change {
        n1960 = event-data() -> ()  [unwired: 7 out]
        n1961 = flat-sequence {
          frame #0 {
            n1962 = Multiply(x="Delay to Interlace (s)", y=1000.0) -> (x*y=w3281:dbl)
            n1963 = Wait (ms)(milliseconds to wait=w3281) -> ()  [unwired: 1 out]
          }
          frame #1 {
            n1964 = property on="Green laser mode" class="RadioBtnsControl (strict)"("Val(Sgnl)"=enum32{"Laser ON", "Laser OFF", "Interlace"}."Interlace" ("Value (Signaling)")) -> ()  [unwired: 2 in, 2 out]
          }
        }
      }
      event "BD 1 Amplitude 1 (%)", "BD 1 Amplitude 2 (%)", "BD 1 Amplitude 3 (%)", "BD 2 Amplitude 1 (%)", "BD 2 Amplitude 2 (%)", "BD 2 Amplitude 3 (%)", "Trap 1 ON", "Trap 2 ON", "Trap 3 ON", "Feedback On/Off", "All FB On/Off": Value Change {
        w3305 = i16 1 ("f")
        n1965 = event-data() -> ()  [unwired: 7 out]
        n1966 = local write "Trap 1 (ON/OFF)"("Trap 1 ON") -> ()
        n1967 = local write "Trap 2 (ON/OFF)"("Trap 2 ON") -> ()
        n1968 = Boolean To (0,1)(Boolean="Trap 3 ON") -> (0, 1=w3306:i16)
        n1969 = Boolean To (0,1)(Boolean="Trap 1 ON") -> (0, 1=w3307:i16)
        n1970 = Boolean To (0,1)(Boolean="Trap 2 ON") -> (0, 1=w3308:i16)
        n1971 = Select(t=w3308, s="Trap ON/OFF X or Y Amp?", f=w3305) -> (s? t:f=w3303:i16)
        n1972 = Select(t=w3307, s="Trap ON/OFF X or Y Amp?", f=w3305) -> (s? t:f=w3304:i16)
        n1973 = Select(t=w3306, s="Trap ON/OFF X or Y Amp?", f=w3305) -> (s? t:f=w3302:i16)
        n1974 = Select(t=w3305, s="Trap ON/OFF X or Y Amp?", f=w3308) -> (s? t:f=w3300:i16)
        n1975 = Select(t=w3305, s="Trap ON/OFF X or Y Amp?", f=w3307) -> (s? t:f=w3301:i16)
        n1976 = Select(t=w3305, s="Trap ON/OFF X or Y Amp?", f=w3306) -> (s? t:f=w3299:i16)
        n1977 = And(x="All FB On/Off", y="Feedback On/Off") -> (x .and. y?=w3297:cluster{"Set 1":bool, "Set 2":bool})
        n1978 = local read "BD 1 Amplitude 1 (%)"() -> (w3317:dbl)
        n1979 = local read "BD 1 Amplitude 2 (%)"() -> (w3316:dbl)
        n1980 = local read "BD 1 Amplitude 3 (%)"() -> (w3315:dbl)
        n1981 = Unbundle By Name(w3297) -> ("Set 1"=w3292:bool, "Set 2"=w3289:bool)
        n1982 = local read "Y RF Amplitude Limits (%)"() -> (w3285:T16)
        n1983 = local read "X RF Amplitude Limits (%)"() -> (w3286:T16)
        n1984 = local read "BD 2 Amplitude 1 (%)"() -> (w3318:dbl)
        n1985 = local read "BD 2 Amplitude 2 (%)"() -> (w3319:dbl)
        n1986 = local read "BD 2 Amplitude 3 (%)"() -> (w3320:dbl)
        n1987 = And(x="Trap 2 ON", y=w3289) -> (x .and. y?=w3287:bool)
        n1988 = And(x="Trap 1 ON", y=w3292) -> (x .and. y?=w3290:bool)
        n1989 = Multiply(x=w3304, y=w3317) -> (x*y=w3312:dbl)
        n1990 = Multiply(x=w3316, y=w3303) -> (x*y=w3310:dbl)
        n1991 = Multiply(x=w3315, y=w3302) -> (x*y=w3311:dbl)
        n1992 = Multiply(x=w3318, y=w3301) -> (x*y=w3321:dbl)
        n1993 = Multiply(x=w3319, y=w3300) -> (x*y=w3322:dbl)
        n1994 = Multiply(x=w3320, y=w3299) -> (x*y=w3323:dbl)
        n1995 = call "set RF board amplitude - interlace.vi"("Board 2 Amplitude Limits"=w3285, "Board 1 Amplitude Limits"=w3286, "error in"=w3313, "FPGA VI Reference In"=w3314, "Board 2 Amplitude 3 (%)"=w3323, "Board 1 Amplitude 3 (%)"=w3311, "Board 2 Amplitude 2 (%)"=w3322, "Board 2 Amplitude 1 (%)"=w3321, "Board 1 Amplitude 2 (%)"=w3310, "Board 1 Amplitude 1 (%)"=w3312) -> ("error out"=w3294:errorcluster, "FPGA VI Reference Out"=w3295:T19)
        n1996 = xnode "Read/Write Control"("FPGA VI Reference In"=w3295, "error in"=w3294, "FB On/Off Set 1"=w3290, "FB On/Off Set 2"=w3287) -> ("error out"=w3293:errorcluster)  [unwired: 1 out]
      }
      event "Load parameters": Value Change {
        n1997 = event-data() -> ()  [unwired: 7 out]
        n1998 = property on="Saved AOD Raster Scan Parameter Sets" class="Arr (strict)"() -> ("Index Values"=w3334:u32[])  [unwired: 2 in, 2 out]
        n1999 = Index Array(array=w3334, index=0) -> (element=w3331:u32)
        n2000 = local write "Load parameters"(FALSE ("Load parameters")) -> ()
        n2001 = Index Array(array="Saved AOD Raster Scan Parameter Sets", index=w3331) -> (element=w3330:T43)
        n2002 = Unbundle By Name(w3330) -> ("Scan Range AOD (nm) 2"=w3329:dbl, "Step Size AOD (nm) 2"=w3328:dbl, "Scan Speed AOD (nm/s) 2"=w3327:dbl, "Number of scans (AOD) 2"=w3326:u16)
        n2003 = flat-sequence {
          tunnel: w3329 -> [w3337]
          tunnel: w3328 -> [w3336]
          tunnel: w3327 -> [w3335]
          tunnel: w3326 -> [w3338]
          frame #0 {
            n2004 = local write "Scan Speed (nm/s)"(w3335) -> ()
            n2005 = local write "Scan Range (nm)"(w3337) -> ()
            n2006 = local write "Step Size (nm)"(w3336) -> ()
          }
          frame #1 {
            n2007 = property on="Number of F/B Scans (AOD)" class="DigNum (strict)"("Val(Sgnl)"=w3338) -> ()  [unwired: 2 in, 2 out]
          }
        }
      }
      event "Trap 1 (ON/OFF)", "Trap 2 (ON/OFF)": Value Change {
        n2008 = event-data() -> ()  [unwired: 7 out]
        n2009 = property on="Trap 2 ON" class="Bool (strict)"("Val(Sgnl)"="Trap 2 (ON/OFF)") -> ()  [unwired: 2 in, 2 out]
        n2010 = property on="Trap 1 ON" class="Bool (strict)"("Val(Sgnl)"="Trap 1 (ON/OFF)") -> ()  [unwired: 2 in, 2 out]
      }
      event "DIO count 1 (ticks)", "DIO count 2 (ticks)", "DIO count 3 (ticks)", "Interlace", "Number Interlace Sets", "Not-Interlacing Set": Value Change {
        n2011 = event-data() -> ()  [unwired: 7 out]
        n2012 = local read "DIO count 3 (ticks)"() -> (w3351:u32)
        n2013 = local read "DIO count 1 (ticks)"() -> (w3353:u32)
        n2014 = local read "DIO count 2 (ticks)"() -> (w3352:u32)
        n2015 = To Unsigned Byte Integer(number="Not-Interlacing Set") -> (unsigned 8bit integer=w3342:u8)
        n2016 = Add(x=w3342, y=u8 1) -> (x+y=w3346:u8)
        n2017 = xnode "Read/Write Control"("FPGA VI Reference In"=w3357, "error in"=w3355, "DIO count 1 (ticks)"=w3353, "DIO count 2 (ticks)"=w3352, "DIO count 3 (ticks)"=w3351, "Interlace ON/OFF"="Interlace", "Number Interlace Cycles"="Number Interlace Sets", "Interlace Off Parameters"=w3346) -> ("error out"=w3356:errorcluster)  [unwired: 1 out]
        n2018 = Build Array(w3353, w3352, w3351) -> (w3344:u32[])
        n2019 = Split 1D Array(array=w3344, index="Number Interlace Sets") -> (first subarray=w3354:u32[])  [unwired: 1 out]
        n2020 = Index Array(array=w3344, index=w3342) -> (element=w3343:u32)
        n2021 = Add Array Elements(numeric array=w3354) -> (sum=w3348:u32)
        n2022 = Select(t=w3348, s="Interlace", f=w3343) -> (s? t:f=→"Total Counts (ticks)":u32)
      }
      event "Reset Feedback": Value Change {
        n2023 = event-data() -> ()  [unwired: 7 out]
        n2024 = Unbundle By Name("Reset Feedback") -> ("Set 1"=w3361:bool, "Set 2"=w3360:bool)
        n2025 = xnode "Read/Write Control"("FPGA VI Reference In"=w3363, "error in"=w3358, "FB Reset Set 1"=w3361, "FB Reset Set 2"=w3360) -> ("error out"=w3359:errorcluster)  [unwired: 1 out]
      }
      event "PID Gains": Value Change {
        n2026 = event-data() -> ()  [unwired: 7 out]
        n2027 = Unbundle By Name("PID Gains") -> ("Set 1"=w3367:T14, "Set 2"=w3366:T14)
        n2028 = xnode "Read/Write Control"("FPGA VI Reference In"=w3368, "error in"=w3364, "FB Gains Set 1"=w3367, "FB Gains Set 2"=w3366) -> ("error out"=w3365:errorcluster)  [unwired: 1 out]
      }
      event "AI2 to Setpoint", "Setpoints (V)": Value Change {
        n2029 = event-data() -> ()  [unwired: 7 out]
        n2030 = xnode "Read/Write Control"("FPGA VI Reference In"=w3374, "error in"=w3370) -> ("FPGA VI Reference Out"=w3373:T19, "error out"=w3372:errorcluster, "AI2 Y Sum Set 1"=w3381:i16, "AI2 Y Sum Set 2"=w3380:i16)
        n2031 = Cluster To Array(cluster="AI2 to Setpoint") -> (array=w3384:bool[])
        n2032 = local read "AI2 (V)"() -> (w3382:cluster{"Set 1":dbl, "Set 2":dbl})
        n2033 = Or Array Elements(Boolean array=w3384) -> (logical OR=w3385:bool)
        n2034 = Bundle By Name(cluster=w3382, "Set 1"=w3381, "Set 2"=w3380) -> (w3379:cluster{"Set 1":dbl, "Set 2":dbl})
        n2035 = Divide(x=w3379, y=3276.7) -> (x/y=w3378:cluster{"Set 1":dbl, "Set 2":dbl})
        "AI2 (V)" <- w3378
        n2036 = case shown="True" w3385 {
          tunnel: [w3388 w3405] -> w3377
          tunnel: "AI2 to Setpoint" -> [_ w3401]
          tunnel: "Setpoints (V)" -> [w3389 w3404]
          tunnel: w3378 -> [_ w3398]
          frame False {
            n2037 = Multiply(x=3276.7, y=w3389) -> (x*y=w3390:cluster{"Set 1":dbl, "Set 2":dbl})
            n2038 = To Word Integer(number=w3390) -> (16bit integer=w3388:cluster{"Set 1":i16, "Set 2":i16})
          }
          frame True {
            n2039 = Unbundle By Name(w3398) -> ("Set 1"=w3397:dbl, "Set 2"=w3396:dbl)
